vi "get SystemTimeOffset.vi"() -> (2 "UTC Offset":T1=enum."UTC+00:00")   [LabVIEW 2013, in "Epoch.lvclass"]
uses:
  Epoch.lvclass
  UTC Offsets -- enum.ctl
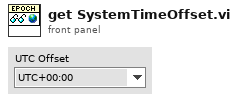
[diagram p1: front panel]
types:
  T1 = typedef "Epoch.lvclass/UTC Offsets -- enum.ctl" = enum16{"UTC-12:00", "UTC-11:00", "UTC-10:00", "UTC-09:30", "UTC-09:00", "UTC-08:00", "UTC-07:00", "UTC-06:00", "UTC-05:00", "UTC-04:00", "UTC-03:30", "UTC-03:00", "UTC-02:00", "UTC-01:00", "UTC+00:00", "UTC+01:00", "UTC+02:00", "UTC+03:00", "UTC+03:30", "UTC+04:00", "UTC+04:30", "UTC+05:00", "UTC+05:30", "UTC+05:45", "UTC+06:00", "UTC+06:30", "UTC+07:00", "UTC+08:00", "UTC+08:45", "UTC+09:00", "UTC+09:30", "UTC+10:00", "UTC+10:30", "UTC+11:00", "UTC+12:00", "UTC+12:45", "UTC+13:00", "UTC+14:00"}
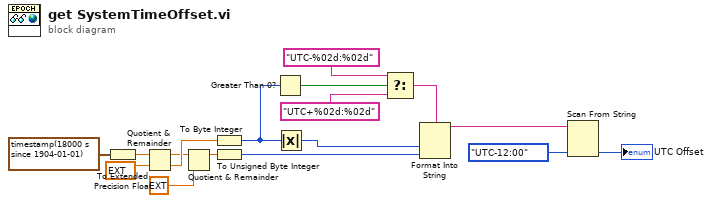
[diagram p0: block diagram]
diagram:
  n1 = To Extended Precision Float(1:timestamp(18000 s since 1904-01-01) ("Timestamp")) -> (0:w2:ext)
  n2 = Quotient & Remainder(x=w2, y=ext 3600.0) -> (x-y*floor(x/y)=w3:ext, floor(x/y)=w14:ext)
  n3 = Quotient & Remainder(x=w3, y=ext 60.0) -> (x-y*floor(x/y)=w15:ext)  [unwired: 1 out]
  n4 = To Byte Integer(number=w14) -> (8bit integer=w5:i8)
  n5 = To Unsigned Byte Integer(number=w15) -> (unsigned 8bit integer=w13:u8)
  n6 = Greater Than 0?(x=w5) -> (x > 0?=w9:bool)
  n7 = Absolute Value(x=w5) -> (abs(x)=w4:i8)
  n8 = Select(t="UTC-%02d:%02d" ("format string"), s=w9, f="UTC+%02d:%02d" ("format string")) -> (s? t:f=w7:string)
  n9 = Format Into String(format string=w7, w4, w13) -> (resulting string=w12:string)  [unwired: 2 in, 1 out]
  n10 = Scan From String(input string=w12, default 1=UTC_Offsets_--_enum."UTC-12:00" ("UTC Time Offset")) -> (output 1=→"UTC Offset":T1)  [unwired: 3 in, 3 out]
